vi "Boolean F-I Test.vi"() -> ()   [LabVIEW 2021]
uses:
  Source/Fault-Injection Bus/Support/Boolean/Support/Value Type.ctl
  Source/Omni-Bus/Omni_Bus.lvclass
  Source/Omni-Bus/Support/Broad Types.ctl
  Source/Local Bus/Local Bus.lvclass
  C:/Users/Tim/Documents/GitHub/Omni-Bus/Source/Omni-Bus/Bus Access/Bus_Access.lvclass
  <vilib>/Utility/Data Type/Type Definitions/Data Type.ctl
  Source/Fault-Injection Bus/Fault-Injection Bus.lvclass
  Source/Omni-Bus/Support/Get/Static/Get Static Boolean.vi
  <vilib>/TSA/Abstract Data Classes/Abs_Types/Boolean/Static Read.vi
  <vilib>/TSA/Abstract Data Classes/Abs_Types/Boolean/Static Write.vi
  <vilib>/TSA/Abstract Data Classes/Abs_Types/Boolean/Abs_Boolean.lvclass
  <vilib>/Utility/Data Type/NI_Data Type.lvlib
  Source/Fault-Injection Bus/Support/Boolean/Fault-Injection_Boolean.lvclass
panel:
  in  "Tag 4":string(combo)
  in  "Boolean":bool
  out "error out 4":errorcluster
  in  "Enable":bool
  in  "Value":T1
  in  "Tag 3":string(combo)
  in  "Arm":bool
  in  "Array":bool[](array[boolean])
  out "Booleans":bool[](array[boolean])
  out "error out 3":errorcluster
  out "error out 2":errorcluster
  in  "Tag 2":string[](array[combo])
  in  "stop":bool
  in  "Tags":string[](array[combo])
  out "error out":errorcluster
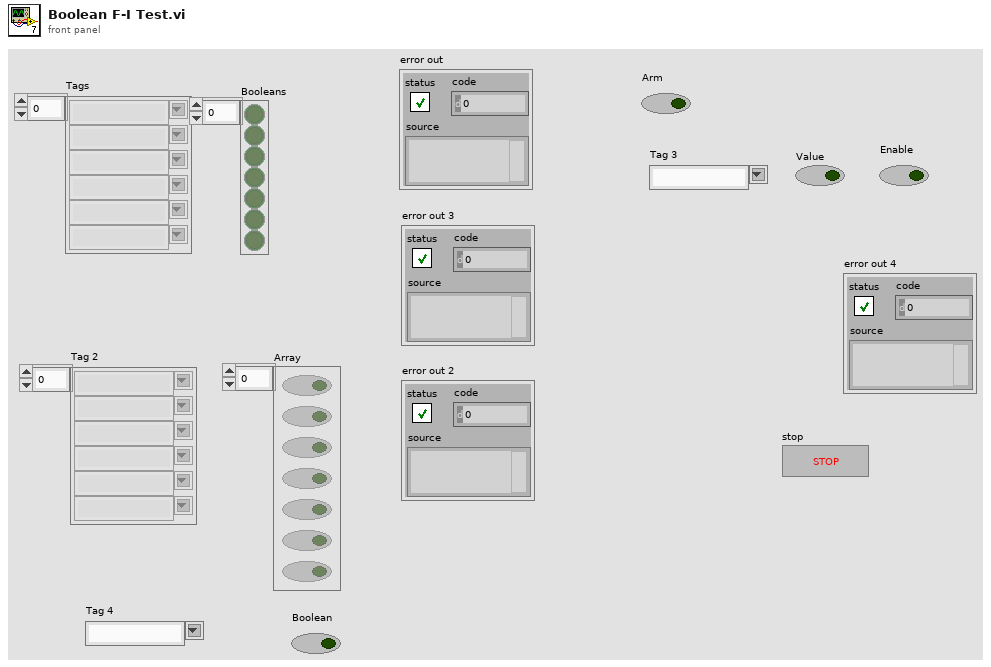
[diagram p1: front panel]
types:
  T1 = typedef "Fault-Injection_Boolean.lvclass/Value Type.ctl" = bool
  T2 = typedef "NI_Data Type.lvlib/Data Type.ctl" = enum8{"Invalid Type", "Void", "I8", "I16", "I32", "I64", "U8", "U16", "U32", "U64", "Single Float", "Double Float", "Extended Float", "Single Complex", "Double Complex", "Extended Complex", "Enum U8", "Enum U16", "Enum U32", "Enum U64", "Single Float With Unit", "Double Float With Unit", "Extended Float With Unit", "Single Complex with Unit", "Double Complex with Unit", "Extended Complex with Unit", "Boolean", "String", "Path", "Picture", "Tag", "Array", "Cluster", "Variant", "LV Variant", "Waveform", "Timestamp", "Digital Waveform", "Digital Data", "ExpressData", "Refnum", "External Data", "VI", "Poly VI", "LabVIEW Class Instance", "Fixed Point", "Set Collection", "Map Collection"}
  T3 = typedef "Omni_Bus.lvclass/Broad Types.ctl" = enum16{"All Tags", "NI Specific Type", "Boolean", "String", "Numeric", "Float", "Integer", "Collection", "All Value Types", "Non Value Types"}
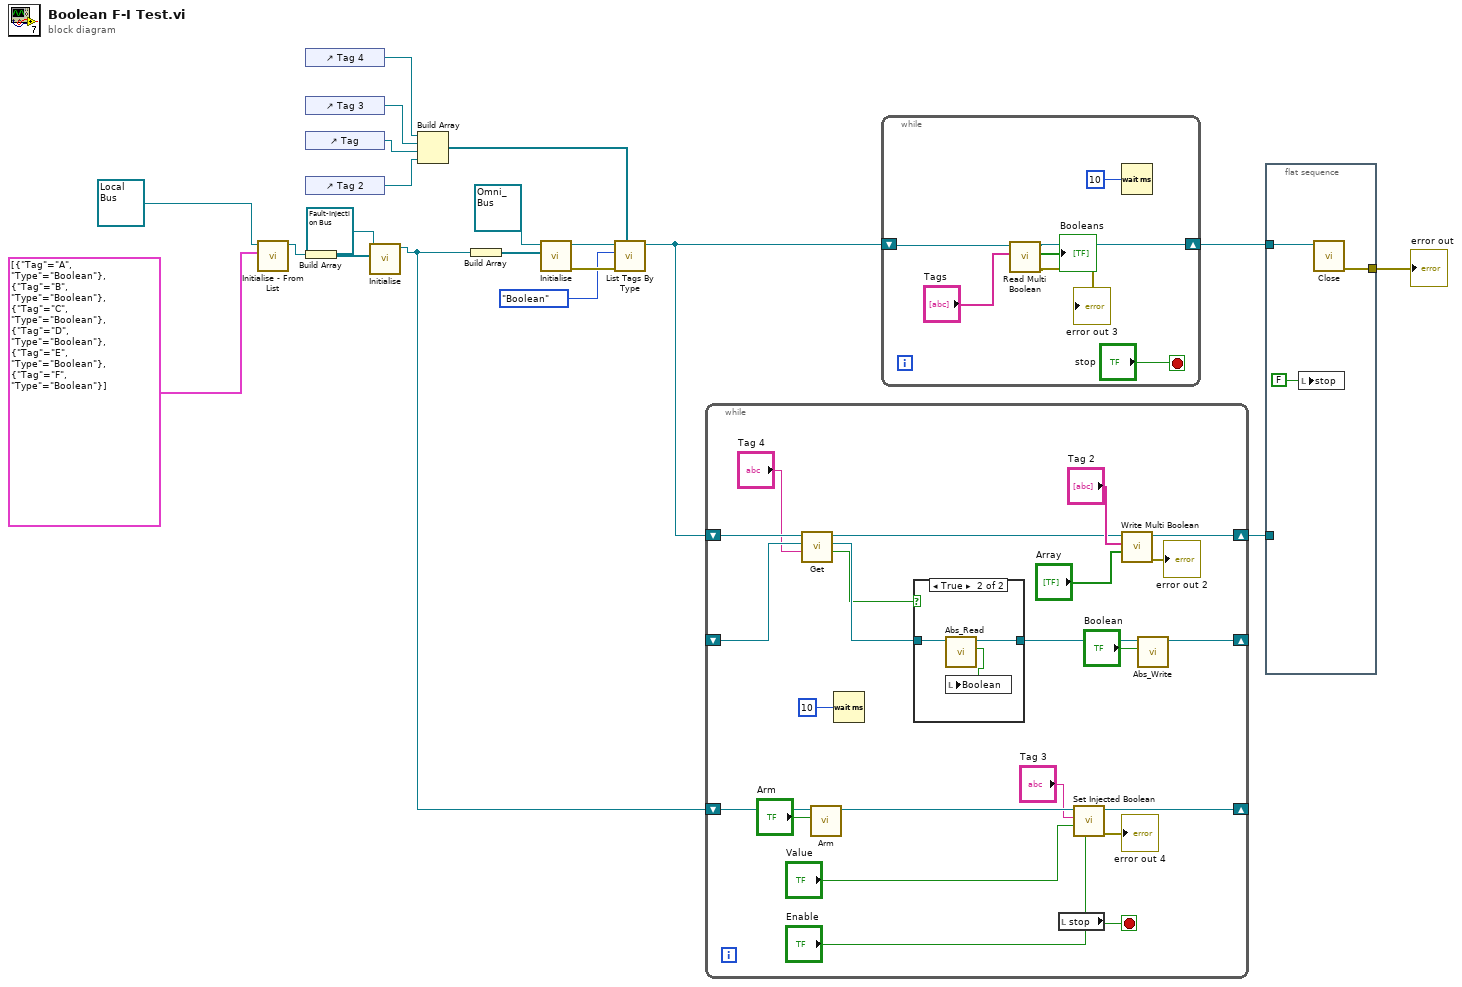
[diagram p0: block diagram]
diagram:
  n1 = call "Initialise - From List.vi"("Tag List"=cluster{"Tag":string, "Type":T2}[] [{"Tag"="A", "Type"=enum."Boolean"}, {"Tag"="B", "Type"=enum."Boolean"}, {"Tag"="C", "Type"=enum."Boolean"}, {"Tag"="D", "Type"=enum."Boolean"}, {"Tag"="E", "Type"=enum."Boolean"}, {"Tag"="F", "Type"=enum."Boolean"}], "Local Bus in"=refnum<class "Local Bus.lvclass"> refnum ("Local Bus.lvclass")) -> ("Local Bus out"=w6:refnum<class "Local Bus.lvclass">)  [unwired: 8 in, 1 out]
  n2 = control-ref of="Tag 4"() -> (w1:refnum<vi>)
  n3 = control-ref of="Tag 3"() -> (w2:refnum<vi>)
  n4 = control-ref of="Tag"() -> (w9:refnum<vi>)
  n5 = control-ref of="Tag 2"() -> (w8:refnum<vi>)
  n6 = Build Array(w6) -> (w5:refnum<class "Local Bus.lvclass">[])
  n7 = call "Initialise.vi"("Buses"=w5, "Fault-Injection Bus in"=refnum<class "Fault-Injection Bus.lvclass"> refnum) -> ("Fault-Injection Bus out"=w3:refnum<class "Fault-Injection Bus.lvclass">)  [unwired: 8 in, 1 out]
  n8 = Build Array(w1, w2, w9, w8) -> (w7:refnum<vi>[])
  n9 = Build Array(w3) -> (w19:refnum<class "Fault-Injection Bus.lvclass">[])
  n10 = call-dynamic "Initialise.vi"("Bus Access"=w19, "Var Bus in"=refnum<class "Omni_Bus.lvclass"> refnum) -> ("error out"=w17:errorcluster, "Var Bus out"=w18:refnum<class "Omni_Bus.lvclass">)  [unwired: 8 in]
  n11 = call-dynamic "List Tags By Type.vi"("Combo Boxes"=w7, "error in (no error)"=w17, "Broad Types"=Broad_Types."Boolean", "Var Bus in"=w18) -> ("Var Bus out"=w13:refnum<class "Omni_Bus.lvclass">)  [unwired: 4 in, 3 out]
  n12 = while {
    shift-right: [w41] -> w12
    shift-left: w13 -> [w29]
    shift-right: [w34] -> _
    shift-left: w3 -> [w37]
    shift-right: [w24] -> _
    shift-left: _ -> [w27]
    stop <- w43 stop-if-true
    n13 = call-poly "Get.vi"("Tag"="Tag 4", "Value Type"=w27, "Var Bus in"=w29) -> ("Updated Tag"=w21:bool, "Value Out"=w26:refnum<class "Abs_Boolean.lvclass">, "Var Bus out"=w28:refnum<class "Omni_Bus.lvclass">)  [unwired: 5 in, 1 out]
    n14 = call "Arm.vi"("Arm"="Arm", "Fault-Injection Bus in"=w37) -> ("Fault-Injection Bus out"=w35:refnum<class "Fault-Injection Bus.lvclass">)  [unwired: 8 in, 1 out]
    n15 = Wait (ms)(milliseconds to wait=u32 10) -> ()  [unwired: 1 out]
    n16 = case shown="True" w21 {
      tunnel: w26 -> [w44 w47]
      tunnel: [w44 w46] -> w25
      frame False {
      }
      frame True {
        n17 = call-poly <vilib>:"Abs_Read.vi"("Abs_Boolean in"=w47) -> ("Boolean"=w45:bool, "Abs_Boolean out"=w46:refnum<class "Abs_Boolean.lvclass">)  [unwired: 8 in, 1 out]
        n18 = local write "Boolean"(w45) -> ()
      }
    }
    n19 = local read "stop"() -> (w43:bool)
    n20 = call "Set Injected Boolean.vi"("Enable"="Enable", "Value"="Value", "Tag"="Tag 3", "Fault-Injection Bus in"=w35) -> ("error out"=→"error out 4":errorcluster, "Fault-Injection Bus out"=w34:refnum<class "Fault-Injection Bus.lvclass">)  [unwired: 6 in]
    n21 = call "Write Multi Boolean.vi"("Array"="Array", "Tag"="Tag 2", "Omni_Bus in"=w28) -> ("error out"=→"error out 2":errorcluster, "Omni_Bus out"=w41:refnum<class "Omni_Bus.lvclass">)  [unwired: 7 in]
    n22 = call-poly <vilib>:"Abs_Write.vi"("Boolean"="Boolean", "Abs_Boolean in"=w25) -> ("Abs_Boolean out"=w24:refnum<class "Abs_Boolean.lvclass">)  [unwired: 8 in, 1 out]
  }
  n23 = while {
    shift-right: [w52] -> w14
    shift-left: w13 -> [w51]
    stop <- "stop" stop-if-true
    n24 = call "Read Multi Boolean.vi"("Tags"="Tags", "Var Bus in"=w51) -> ("error out"=→"error out 3":errorcluster, "Booleans"=→"Booleans":bool[], "Var Bus out"=w52:refnum<class "Omni_Bus.lvclass">)  [unwired: 7 in]
    n25 = Wait (ms)(milliseconds to wait=u32 10) -> ()  [unwired: 1 out]
  }
  n26 = flat-sequence {
    tunnel: [w57] -> w15
    tunnel: w14 -> [w56]
    tunnel: w12 -> [_]
    frame #0 {
      n27 = local write "stop"(FALSE ("stop")) -> ()
      n28 = call-dynamic "Close.vi"("Data in"=w56) -> ("error out"=w57:errorcluster)  [unwired: 9 in, 1 out]
    }
  }
  "error out" <- w15
